vi "Set - Keep Specific Signals Delete the Rest.vi"(0 "reference in":refnum<class "GSwFormDSP.lvclass">, 5 "error in (no error)":errorcluster, 7 "Channels Index to KEEP":i32[](array[numeric])) -> (14 "reference in":refnum<class "GSwFormDSP.lvclass">, 19 "error out":errorcluster)   [LabVIEW 2022 SP3, in "GSwFormDSP.lvclass"]
uses:
  GSwFormDSP.lvclass
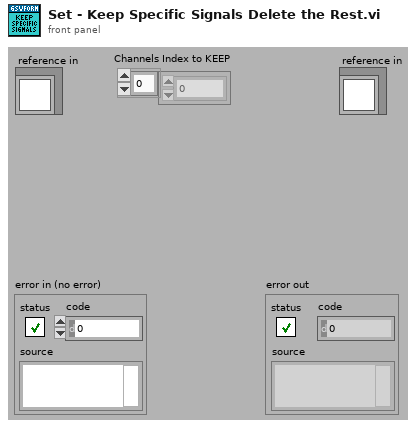
[diagram p1: front panel]
types:
  T1 = typedef "GSwFormDSP.lvclass/ObjectAttributesRef.ctl" = refnum<data-value>
  T2 = typedef "GSwFormDSP.lvclass/ObjectAttributes.ctl" = cluster{"Wform Ref":refnum<data-value>, "Nb Signals":i32, "Spectral Function Parameters":T3, "FFT":waveform(cdb)[], "Nb FFT":i32, "Nb Averages":i32[], "Reference Indexes":i32[], "Response Indexes":i32[], "Coherence":waveform(dbl)[], "TDF Parameters":T5, "DAQ":cluster{"Duration (sec)":dbl, "Buffer Size (Samples)":i32, "Offset (Samples)":i32}, "Filter Impulse Response (TDF)":waveform(dbl), "Sound Playback":T6}
  T3 = typedef "GSwFormDSP.lvclass/Spectral Parameters.ctl" = cluster{"Frequency resolution (Hz)":dbl, "Overlap":dbl, "Window":T4}
  T4 = typedef "NI_AALPro.lvlib/windowTd.ctl" = u32
  T5 = typedef "GSwFormDSP.lvclass/TDF Parameters.ctl" = cluster{"Filter":enum32{"Lowpass", "Highpass", "Bandpass", "Bandstop"}, "Type:":enum16{"Butterworth", "Chebyshev", "Inv Chebyshev", "Elliptic", "Bessel"}, "LP cutoff freq":dbl, "HP cutoff freq":dbl, "Order":i32, "passband ripple (dB)":dbl, "stopband attenuation (dB)":dbl, "Phaseless Filter":bool, "Include Fade IN and OUT":bool}
  T6 = typedef "GSwFormDSP.lvclass/Sound Playback.ctl" = cluster{"Timer start (ms)":u32, "task ID":T7, "Cursor Init Location (s)":dbl, "SC Volume":dbl}
  T7 = typedef "Sound Output Task ID.ctl" = u32
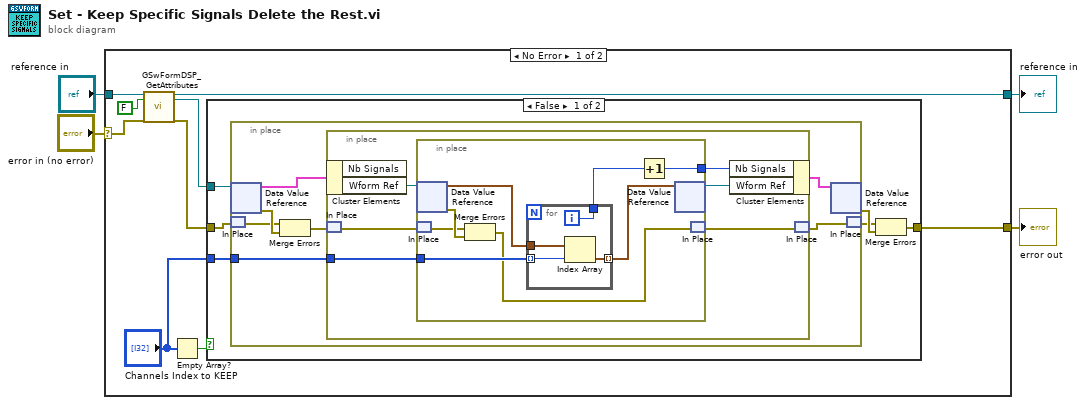
[diagram p0: block diagram]
diagram:
  n1 = case shown="No Error" "error in (no error)" {
    selector: "error in (no error)" -> [w10 w47]
    tunnel: [w13 w47] -> w3
    tunnel: [w7 w46] -> w1
    tunnel: "reference in" -> [w8 w46]
    frame No Error {
      n2 = call "GSwFormDSP_GetAttributes.vi"("reference in"=w8, "return data? (T)"=FALSE, "error in (no error)"=w10) -> ("reference out"=w7:refnum<class "GSwFormDSP.lvclass">, "attributes ref"=w6:T1, "error out"=w5:errorcluster)  [unwired: 13 in, 1 out]
      n3 = Empty Array?(array="Channels Index to KEEP") -> (empty?=w12:bool)
      n4 = case shown="False" w12 {
        tunnel: [w19 w45] -> w13
        tunnel: "Channels Index to KEEP" -> [w18 _]
        tunnel: w6 -> [w16 _]
        tunnel: w5 -> [w15 w45]
        frame False {
          n5 = in-place {
            in-place-border: w18 -> [w26]
            n6 = in-place-dvr #1(w16) -> (w23:T2, w25:errorcluster)
            n7 = in-place-match #2(w15) -> (w24:errorcluster)
            n8 = Merge Errors(w24, w25) -> (w21:errorcluster)
            n9 = in-place {
              in-place-border: w26 -> [w32]
              n10 = in-place-cluster #3(w23) -> ("Wform Ref"=w31:refnum<data-value>)  [unwired: 1 out]
              n11 = in-place-match #4(w21) -> (w30:errorcluster)
              n12 = in-place {
                in-place-border: w32 -> [w40]
                in-place-border: [w33] -> w27
                n13 = in-place-dvr #5(w31) -> (w37:waveform(dbl)[], w39:errorcluster)
                n14 = in-place-match #6(w30) -> (w38:errorcluster)
                n15 = Merge Errors(w38, w39) -> (w35:errorcluster)
                n16 = for {
                  tunnel: w40 -> [w44] mode=indexing
                  tunnel: [w43] -> w36 mode=indexing
                  tunnel: w37 -> [w42]
                  tunnel: [w41] -> w34
                  i -> [w41]
                  n17 = Index Array(array=w42, index=w44) -> (element=w43:waveform(dbl))
                }
                n18 = Increment(x=w34) -> (x+1=w33:i32)
                n19 = in-place-dvr #5(w36) -> (w29:refnum<data-value>)  [unwired: 1 out]
                n20 = in-place-match #6(w35) -> (w28:errorcluster)
              }
              n21 = in-place-cluster #3("Nb Signals"=w27, "Wform Ref"=w29) -> (w22:T2)
              n22 = in-place-match #4(w28) -> (w20:errorcluster)
            }
            n23 = in-place-dvr #1(w22) -> (w17:errorcluster)  [unwired: 1 out]
            n24 = in-place-match #2(w20) -> (w14:errorcluster)
          }
          n25 = Merge Errors(w14, w17) -> (w19:errorcluster)
        }
        frame True {
          # "No Channels were specified, so do nothing!!"
        }
      }
    }
    frame Error {
    }
  }
  "error out" <- w3
  "reference in" <- w1
